vi "TotalDist.vi"(11 "Path":T1=[{"X"=0.0, "Y"=0.0, "OnOff"=TRUE}, {"X"=0.0, "Y"=0.5, "OnOff"=TRUE}, {"X"=0.5, "Y"=1.0, "OnOff"=TRUE}, {"X"=1.0, "Y"=0.5, "OnOff"=TRUE}, {"X"=0.5, "Y"=0.0, "OnOff"=TRUE}, {"X"=0.0, "Y"=0.5, "OnOff"=TRUE}, {"X"=0.0, "Y"=0.0, "OnOff"=TRUE}]) -> (3 "TotalDistance":dbl)   [LabVIEW 2014]
uses:
  Path.ctl
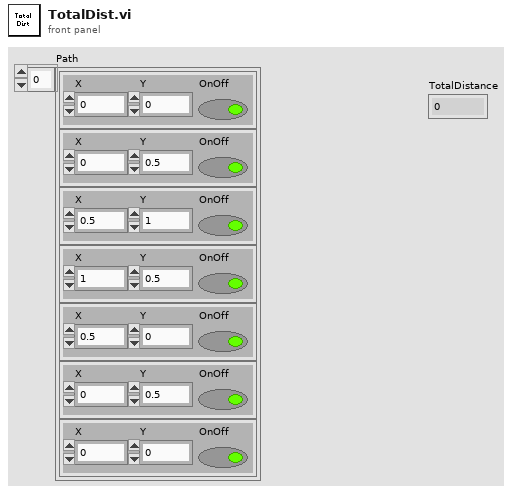
[diagram p1: front panel]
types:
  T1 = typedef "Path.ctl" = cluster{"X":dbl, "Y":dbl, "OnOff":bool}[]
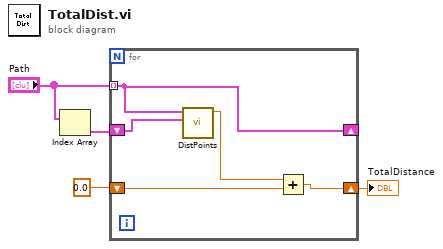
[diagram p0: block diagram]
diagram:
  n1 = Index Array(array="Path") -> (element=w3:cluster{"X":dbl, "Y":dbl, "OnOff":bool})  [unwired: 1 in]
  n2 = for {
    tunnel: "Path" -> [w8] mode=indexing
    shift-right: [w8] -> _
    shift-left: w3 -> [w9]
    shift-right: [w5] -> w1
    shift-left: 0.0 -> [w7]
    n3 = call "DistPoints.vi"("Point2"=w9, "Point1"=w8) -> ("Distance"=w6:dbl)  [unwired: 9 in]
    n4 = Add(x=w6, y=w7) -> (x+y=w5:dbl)
  }
  "TotalDistance" <- w1
